vi "Read Limit Test Result.vi"(5 "Auto Null Offset For Limit Test(F: Disable)":bool, 6 "Limit Test Data Size (0)":i32, 7 "Limit Test Data Offset (0)":i32, 8 "error in (no error)":errorcluster, 10 "Channel (0: Channel 1)":i32(ring) items=["Channel 1", "Channel 2"], 11 "VISA resource name":refnum<visa-resource-name>) -> (0 "error out":errorcluster, 1 "Limit Test Data":T1, 2 "Limit Test Failed?":bool[](array[boolean]), 3 "VISA resource name out":refnum<visa-resource-name>)   [LabVIEW 2020, in "Agilent B2900 Series.lvlib"]
doc: "Calculating the limit test data. The limit test means a pass/fail judgement performed while a composite limit test.\n\n<B>Note:</B>\nCommands in default part of the case structure are not applicable for Agilent models B2961A,B2962A, B2961B and B2962B"
uses:
  Agilent B2900 Series.lvlib
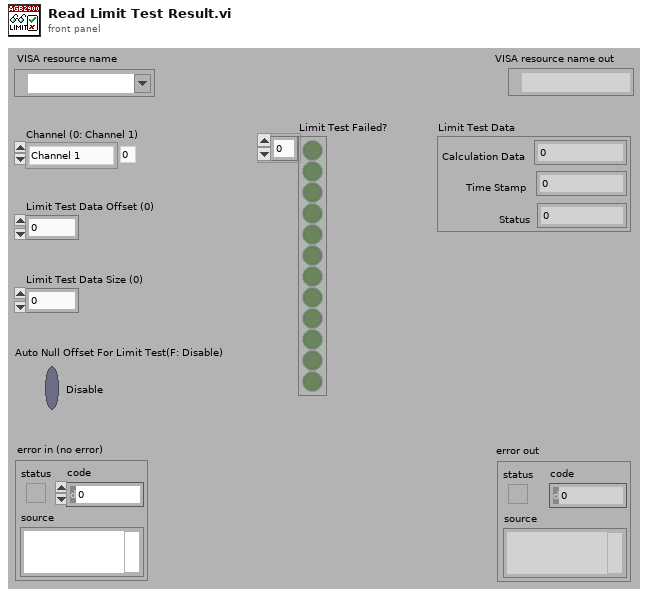
[diagram p1: front panel]
types:
  T1 = cluster{"Calculation Data":dbl, "Time Stamp":dbl, "Status":dbl}
  T2 = typedef "Agilent B2900 Series.lvlib/Extended User Data.ctl" = cluster{"B2900 Series Mode":u16}
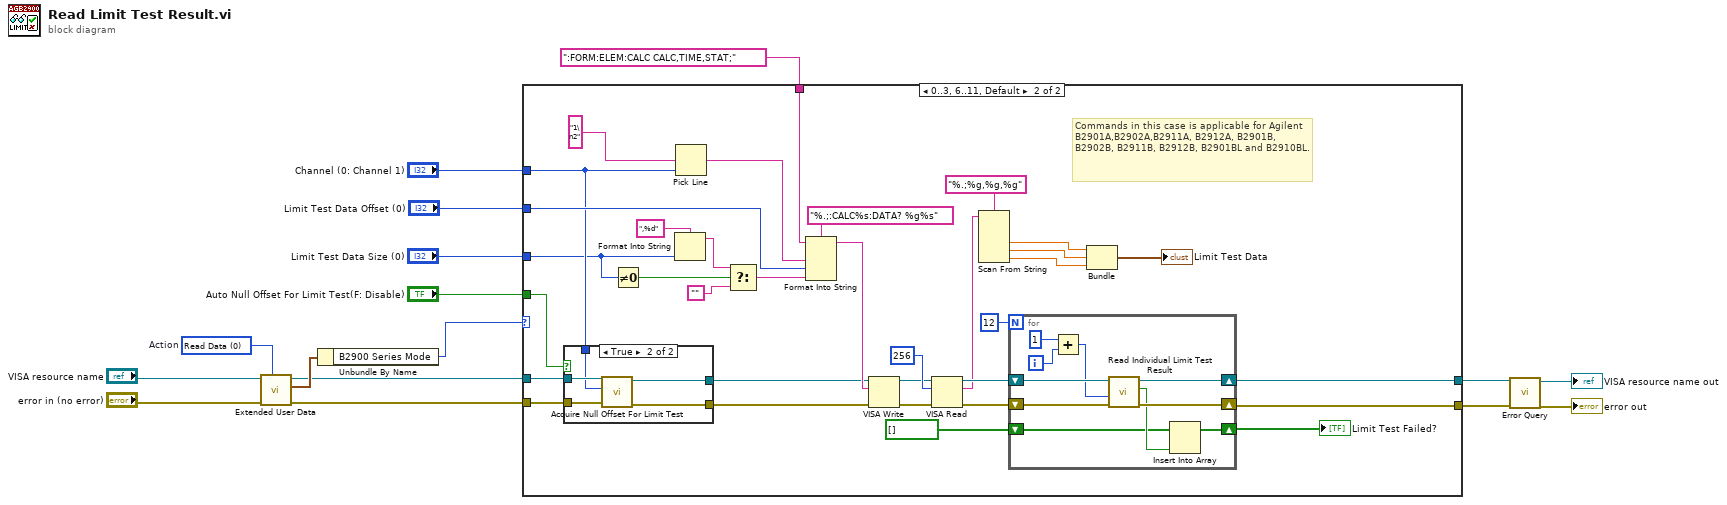
[diagram p0: block diagram]
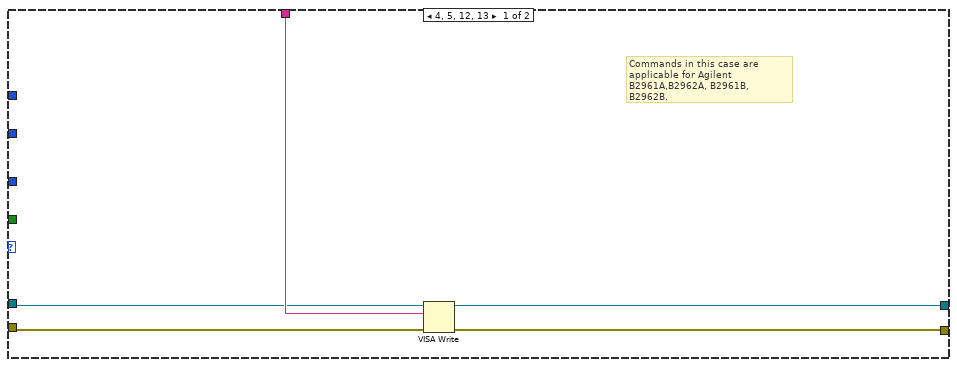
[diagram p2: hidden frame]
diagram:
  w14 = 0 items=["Read Data", "Write Data", "Clear Data", "Clear ALL Data"]  # Action
  n1 = call "Extended User Data.vi"("Action (1: Write Data)"=w14, "Error In (no error)"="error in (no error)", "VISA resource name in"="VISA resource name") -> ("Error Out"=w3:errorcluster, "User Data Out"=w13:T2, "VISA resource name out"=w4:refnum<visa-resource-name>)  [unwired: 6 in]
  n2 = Unbundle By Name(w13) -> ("B2900 Series Mode"=w10:u16)
  n3 = case shown="0..3, 6..11, Default" w10 {
    tunnel: "Channel (0: Channel 1)" -> [_ w25]
    tunnel: "Auto Null Offset For Limit Test(F: Disable)" -> [_ w31]
    tunnel: "Limit Test Data Size (0)" -> [_ w22]
    tunnel: "Limit Test Data Offset (0)" -> [_ w30]
    tunnel: [w18 w28] -> w5
    tunnel: w4 -> [w20 w27]
    tunnel: w3 -> [w19 w26]
    tunnel: ":FORM:ELEM:CALC CALC,TIME,STAT;" -> [w21 w24]
    tunnel: [w17 w23] -> w1
    frame 4, 5, 12, 13 {
      # "Commands in this case are\napplicable for Agilent B2961A,B2962A, B2961B, B2962B."
      n4 = VISA Write(VISA resource name=w20, write buffer=w21, error in (no error)=w19) -> (VISA resource name out=w18:refnum<visa-resource-name>, error out=w17:errorcluster)  [unwired: 1 out]
    }
    frame 0..3, 6..11, Default {
      # "Commands in this case is applicable for Agilent B2901A,B2902A,B2911A, B2912A, B2901B, B2902B, B2911B, B2912B, B2901BL and B2910BL."
      n5 = case shown="True" w31 {
        tunnel: [w67 w72] -> w32
        tunnel: [w66 w71] -> w33
        tunnel: w27 -> [w67 w70]
        tunnel: w26 -> [w66 w69]
        tunnel: w25 -> [_ w68]
        frame False {
        }
        frame True {
          n6 = call "Acquire Null Offset For Limit Test.vi"("error in (no error)"=w69, "Channel (0: Channel 1)"=w68, "VISA resource name"=w70) -> ("error out"=w71:errorcluster, "VISA resource name out"=w72:refnum<visa-resource-name>)  [unwired: 6 in, 1 out]
        }
      }
      n7 = Not Equal To 0?(x=w22) -> (x != 0?=w39:bool)
      n8 = Format Into String(format string=",%d", w22) -> (resulting string=w35:string)  [unwired: 2 in, 1 out]
      n9 = Pick Line(multi-line string="1\n2" ("string (\"\")"), line index=w25) -> (output string=w38:string)  [unwired: 1 in]
      n10 = Select(t=w35, s=w39, f="" ("Empty String Constant")) -> (s? t:f=w41:string)
      n11 = Format Into String(format string="%.;:CALC%s:DATA? %g%s", initial string=w24, w38, w30, w41) -> (resulting string=w42:string)  [unwired: 1 in, 1 out]
      n12 = VISA Write(VISA resource name=w32, write buffer=w42, error in (no error)=w33) -> (VISA resource name out=w43:refnum<visa-resource-name>, error out=w44:errorcluster)  [unwired: 1 out]
      n13 = VISA Read(VISA resource name=w43, byte count=u32 256, error in (no error)=w44) -> (VISA resource name out=w52:refnum<visa-resource-name>, read buffer=w50:string, error out=w51:errorcluster)  [unwired: 1 out]
      n14 = Scan From String(format string="%.;%g,%g,%g", input string=w50) -> (output 1=w48:dbl, output 2=w55:dbl, output 3=w49:dbl)  [unwired: 5 in, 3 out]
      n15 = for {
        N: 12 -> [_]
        shift-right: [w64] -> w28
        shift-left: w52 -> [w62]
        shift-right: [w63] -> w23
        shift-left: w51 -> [w65]
        shift-right: [w57] -> w29
        shift-left: bool[] [] ("array") -> [w56]
        i -> [w61]
        n16 = Add(x=1, y=w61) -> (x+y=w59:i32)
        n17 = call "Read Individual Limit Test Result.vi"("error in (no error)"=w65, "Limit Test Number (1)"=w59, "VISA resource name"=w62) -> ("error out"=w63:errorcluster, "Limit Test Failed?"=w58:bool, "VISA resource name out"=w64:refnum<visa-resource-name>)  [unwired: 6 in]
        n18 = Insert Into Array(array=w56, new element=w58) -> (w57:bool[])  [unwired: 1 in]
      }
      "Limit Test Failed?" <- w29
      n19 = Bundle(w48, w55, w49) -> (→"Limit Test Data":cluster{dbl, dbl, dbl})  [unwired: 1 in]
    }
  }
  n20 = call "Error Query.vi"("error in (no error)"=w1, "VISA resource name"=w5) -> ("error out"=→"error out":errorcluster, "VISA resource name out"=→"VISA resource name out":refnum<visa-resource-name>)  [unwired: 6 in, 2 out]
